vi "Request Value Reference Updates.vi"(8 "error in (no error)":errorcluster, 9 "Datum Type/Initial Value":variant, 10 "Datum Name":string, 11 "IObserver in":refnum<class "IObserver.lvclass">) -> (0 "error out":errorcluster, 1 "ValueReferenceTransport":refnum<class "ValueReferenceTransport.lvclass">, 2 "Subscription Policy":T1, 3 "IObserver out":refnum<class "IObserver.lvclass">)   [LabVIEW 2017, in "IObserver.lvlib" / "IObserver.lvclass"]
doc: "<License>\nCopyright © 2017 Composed Systems, LLC | All rights reserved\nwww.composed.io\n\nAuthor: Ethan Stern <ethan.stern@composed.io>\n\nThis software is provided \"AS IS\" WITHOUT WARRANTIES, either express or implied, AND IS FOR EDUCATIONAL PURPOSES ONLY.\n</License>"
uses:
  IObserver.lvclass
  C:/Program Files (x86)/National Instruments/LabVIEW 2017/vi.lib/ActorFramework/Actor/Actor.lvclass
  IMediator/ISubscriptionPolicy/ISubscriptionPolicy Reference.ctl
  IMediator/ISubscriptionPolicy/ISubscriptionPolicy.lvclass
  Transport/ValueReferenceTransport/ValueReferenceTransport.lvclass
  C:/Git/mva-framework/Framework/IMediator/ITransport/ITransport.lvclass
  <vilib>/ActorFramework/Actor/Actor.lvclass/Actor.ctl
  <vilib>/ActorFramework/Message Enqueuer/Message Enqueuer.lvclass/Message Enqueuer.ctl
  SubscriptionPolicy/ValueChangeSubscription/ValueChangeSubscription.lvclass/ValueChangeSubscription.ctl
  IMediator/SubscriptionRequest/SubscriptionRequest.lvclass/SubscriptionRequest.ctl
  IObserver Messages/Subscribe Msg/Subscribe Msg.lvclass/Subscribe Msg.ctl
  <vilib>/ActorFramework/Message Enqueuer/Init from Existing Queue.vi
  <vilib>/ActorFramework/Message Enqueuer/Enqueue.vi
  SubscriptionPolicy/ValueChangeSubscription/ValueChangeSubscription.lvclass
  C:/Git/mva-framework/Framework/IMediator/ISubscriptionPolicy/ISubscriptionPolicy.lvclass
  IObserver Messages/Subscribe Msg/Subscribe Msg.lvclass
  C:/Program Files (x86)/National Instruments/LabVIEW 2017/vi.lib/ActorFramework/Message/Message.lvclass
  <vilib>/ActorFramework/Message Priority Queue/Priority Enqueue.vi
  <vilib>/ActorFramework/Message Enqueuer/Message Enqueuer.lvclass
  IMediator/SubscriptionRequest/SubscriptionRequest.lvclass
  <vilib>/ActorFramework/Actor/Actor.lvclass
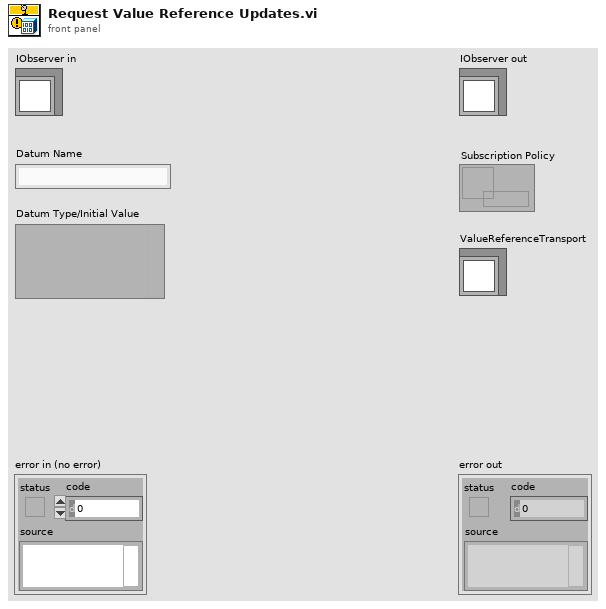
[diagram p1: front panel]
types:
  T1 = typedef "IMediator.lvlib/ISubscriptionPolicy.lvclass/ISubscriptionPolicy Reference.ctl" = refnum<data-value>
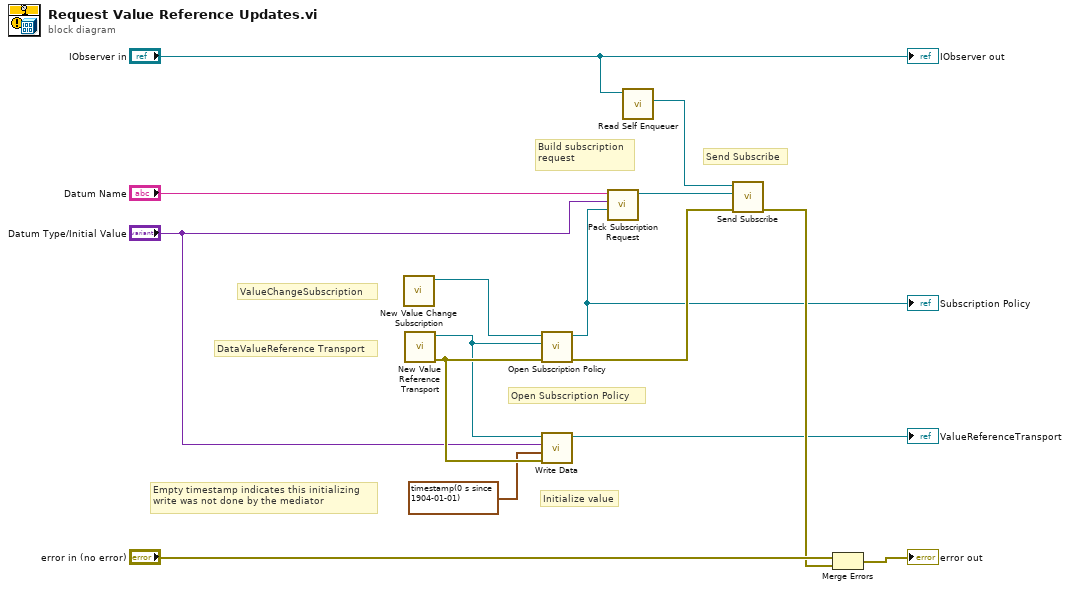
[diagram p0: block diagram]
diagram:
  # "Initialize value"
  # "Empty timestamp indicates this initializing\nwrite was not done by the mediator"
  # "ValueChangeSubscription"
  # "Open Subscription Policy"
  # "Send Subscribe"
  # "Build subscription\nrequest"
  # "DataValueReference Transport"
  n1 = call "New Value Change Subscription.vi"() -> ("ValueChangeSubscription Out"=w13:refnum<class "ValueChangeSubscription.lvclass">)  [unwired: 11 in]
  n2 = call "New Value Reference Transport.vi"() -> ("error out"=w6:errorcluster, "ValueReferenceTransport"=w3:refnum<class "ValueReferenceTransport.lvclass">)  [unwired: 10 in]
  n3 = call "Open Subscription Policy.vi"("error in (no error)"=w6, "Transport"=w3, "SubscriptionPolicy"=w13) -> ("error out"=w9:errorcluster, "Subscription Policy"=w1:T1)  [unwired: 7 in]
  "Subscription Policy" <- w1
  n4 = call-dynamic "Write Data.vi"("error in (no error)"=w6, "Publication Time"=timestamp(0 s since 1904-01-01), "Value"="Datum Type/Initial Value", "ValueReferenceTransport In"=w3) -> ("ValueReferenceTransport Out"=→"ValueReferenceTransport":refnum<class "ValueReferenceTransport.lvclass">)  [unwired: 6 in, 1 out]
  n5 = call "Pack Subscription Request.vi"("Subscription Policy"=w1, "Type"="Datum Type/Initial Value", "Datum Name"="Datum Name") -> ("SubscriptionRequest"=w10:refnum<class "SubscriptionRequest.lvclass">)  [unwired: 8 in]
  n6 = call <vilib>:"Read Self Enqueuer.vi"("Actor"="IObserver in") -> ("Self Enqueuer"=w7:refnum<class "Message Enqueuer.lvclass">)  [unwired: 10 in]
  n7 = call "Send Subscribe.vi"("error in (no error)"=w9, "SubscriptionRequest"=w10, "Message Enqueuer"=w7) -> ("error out"=w8:errorcluster)  [unwired: 7 in, 1 out]
  n8 = Merge Errors("error in (no error)", w8) -> (→"error out":errorcluster)
  "IObserver out" <- "IObserver in"
